vi "setPDTarget.vi"(8 "error in (no error)":errorcluster, 10 "Photodiode Targets":i32[](array[numeric]), 11 "Arduino session":refnum<visa-resource-name>) -> (0 "error out":errorcluster, 3 "Arduino session":refnum<visa-resource-name>)   [LabVIEW 2017]
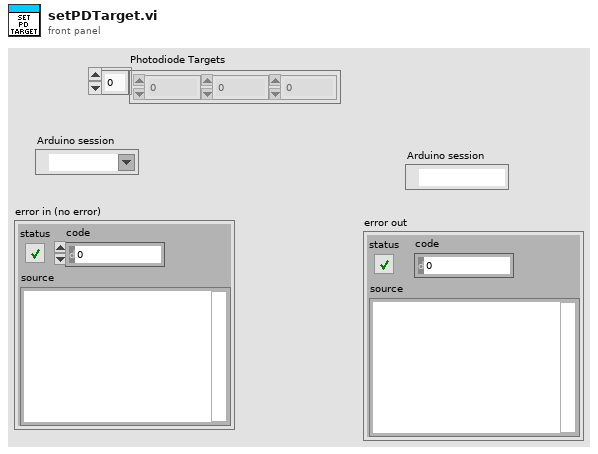
[diagram p1: front panel]
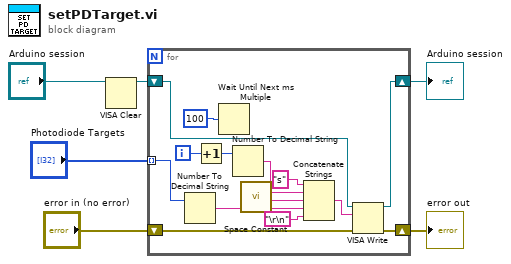
[diagram p0: block diagram]
diagram:
  n1 = VISA Clear(VISA resource name="Arduino session") -> (VISA resource name out=w4:refnum<visa-resource-name>)  [unwired: 1 in, 1 out]
  n2 = for {
    tunnel: "Photodiode Targets" -> [w17] mode=indexing
    shift-right: [w8] -> w2
    shift-left: w4 -> [w18]
    shift-right: [w7] -> w1
    shift-left: "error in (no error)" -> [w19]
    i -> [w16]
    n3 = Number To Decimal String(number=w17) -> (decimal integer string=w11:string)  [unwired: 1 in]
    n4 = Increment(x=w16) -> (x+1=w15:i32)
    n5 = Wait Until Next ms Multiple(millisecond multiple=u32 100) -> ()  [unwired: 1 out]
    n6 = Number To Decimal String(number=w15) -> (decimal integer string=w14:string)  [unwired: 1 in]
    n7 = call <vilib>:"Space Constant.vi"() -> ("String"=w12:string)
    n8 = Concatenate Strings("s" ("string"), w14, w12, w11, "\r\n") -> (w10:string)
    n9 = VISA Write(VISA resource name=w18, write buffer=w10, error in (no error)=w19) -> (VISA resource name out=w8:refnum<visa-resource-name>, error out=w7:errorcluster)  [unwired: 1 out]
  }
  "Arduino session" <- w2
  "error out" <- w1
